vi "Test citire I2C.vi"(0 "bytesToRead":u32=10, 5 "slaveAddress":u8=189 format="%.0b", 9 "use7bitAddress":bool, 11 "error in (no error)":errorcluster) -> (1 "12 bit LSB value (x)":i32, 2 "12 bit LSB value (y)":i32, 3 "12 bit LSB value (z)":i32, 4 "12 bit Field value (mT) X":dbl=0.392, 6 "12 bit Field value (mT) Y":dbl=0.196, 8 "12 bit Field value (mT) Z":dbl=0.098, 10 "12 bit temp (C)":dbl=27.2, 13 "12 bit LSB value (temp)":i32, 14 "FRM":i32=3, 15 "error out":errorcluster)   [LabVIEW 2020]
uses:
  mcp2221_dll_um_x64.dll
panel:
  in  "Tab Control":enum32{"Page 1", "Page 2"}(tab)
  out "noOfDevs out":u32=1
  out "handle out":u64=57196
  out "i2cRxData out":u8[](array[numeric])=[0, 0, 0, 28, 19, 32, 85, 7, 4, 32]
  out "hex integer string":string[](array[string])=["0", "0", "0", "1C", "13", "20", "55", "7", "4", "20"]
  # "I2C Read Config"
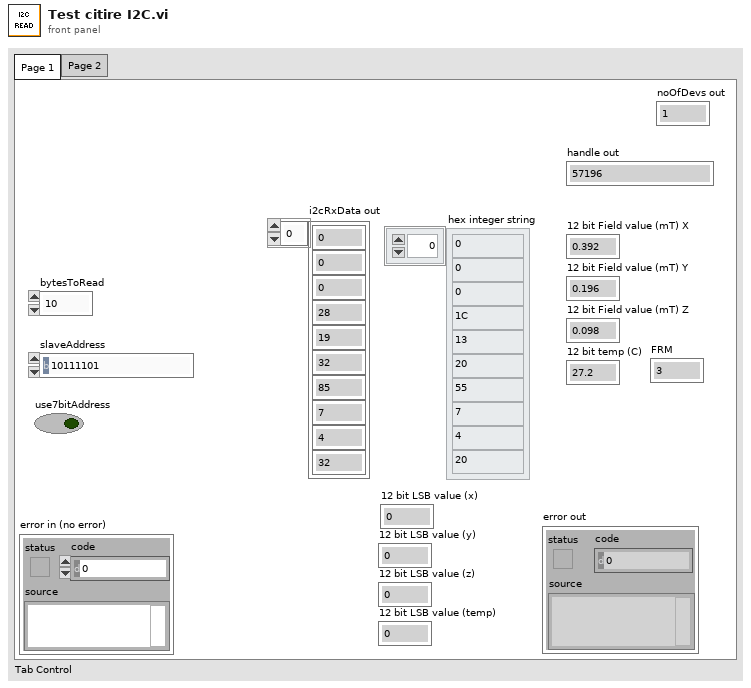
[diagram p1: front panel]
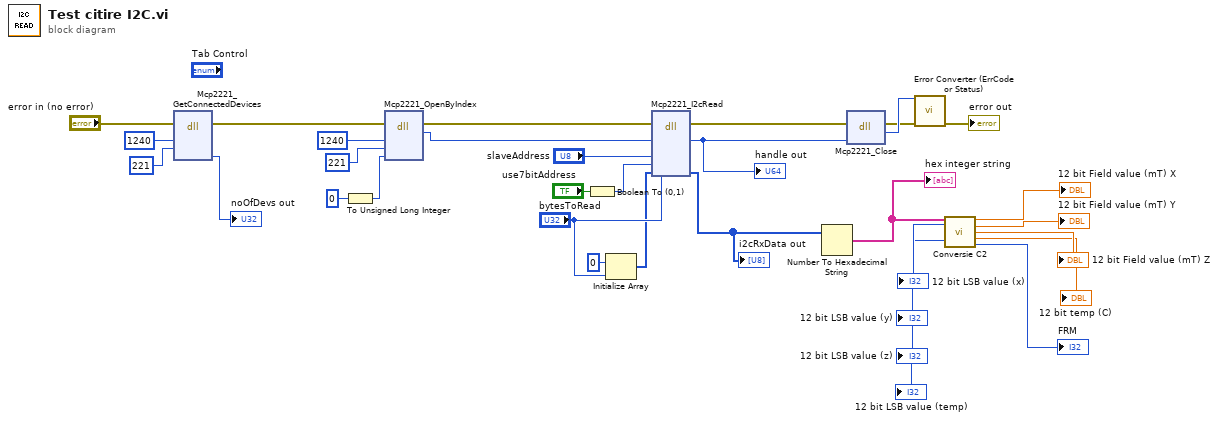
[diagram p0: block diagram]
diagram:
  n1 = dll-call lib="C:/Users/tuguialexand/Desktop/Licenta/MCP2221A LabVIEW library/Microchip MCP2221A_64bit/VIs/Private/mcp2221_dll_um_x64.dll" fn="Mcp2221_GetConnectedDevices"(error in="error in (no error)", "vid"=u32 1240, "pid"=u32 221) -> (error out=w18:errorcluster, "noOfDevs"=→"noOfDevs out":u32)  [unwired: 6 in, 1 out]
  n2 = To Unsigned Long Integer(number=0 ("index")) -> (unsigned 32bit integer=w21:u32)
  n3 = dll-call lib="C:/Users/tuguialexand/Desktop/Licenta/MCP2221A LabVIEW library/Microchip MCP2221A_64bit/VIs/Private/mcp2221_dll_um_x64.dll" fn="Mcp2221_OpenByIndex"(error in=w18, "VID"=u32 1240, "PID"=u32 221, "index"=w21) -> (error out=w16:errorcluster, "return type"=w17:u64)  [unwired: 5 in, 1 out]
  n4 = Boolean To (0,1)(Boolean="use7bitAddress") -> (0, 1=w27:i16)
  n5 = Initialize Array(u8 0, "bytesToRead") -> (w24:u8[])
  n6 = dll-call lib="C:/Users/tuguialexand/Desktop/Licenta/MCP2221A LabVIEW library/Microchip MCP2221A_64bit/VIs/Private/mcp2221_dll_um_x64.dll" fn="Mcp2221_I2cRead"(error in=w16, "handle"=w17, "bytesToRead"="bytesToRead", "slaveAddress"="slaveAddress", "use7bitAddress"=w27, "i2cRxData"=w24) -> (error out=w12:errorcluster, "handle"=w15:u64, "i2cRxData"=w11:u8[])  [unwired: 6 in, 1 out]
  "handle out" <- w15
  "i2cRxData out" <- w11
  n7 = Number To Hexadecimal String(2:w11) -> (0:w10:string[])  [unwired: 1 in]
  "hex integer string" <- w10
  n8 = dll-call lib="C:/Users/tuguialexand/Desktop/Licenta/MCP2221A LabVIEW library/Microchip MCP2221A_64bit/VIs/Private/mcp2221_dll_um_x64.dll" fn="Mcp2221_Close"(error in=w12, "handle"=w15) -> (error out=w13:errorcluster, "return type"=w14:i32)  [unwired: 3 in, 1 out]
  n9 = call "Error Converter (ErrCode or Status).vi"("error code"=w14, "error in (no error)"=w13) -> ("error out"=→"error out":errorcluster)  [unwired: 13 in]
  n10 = call "Conversie C2.vi"("Array"=w10) -> ("12 bit LSB value (x)"=→"12 bit LSB value (x)":i32, "12 bit LSB value (y)"=→"12 bit LSB value (y)":i32, "12 bit LSB value (z)"=→"12 bit LSB value (z)":i32, "12 bit Field value (mT) X"=→"12 bit Field value (mT) X":dbl, "12 bit Field value (mT) Y"=→"12 bit Field value (mT) Y":dbl, "12 bit Field value (mT) Z"=→"12 bit Field value (mT) Z":dbl, "12 bit temp (C)"=→"12 bit temp (C)":dbl, "12 bit LSB value (temp)"=→"12 bit LSB value (temp)":i32, "FRM"=→"FRM":i32)  [unwired: 6 in]
